vi "Test MQTT-3.1.0-1.vi"(8 "error in (no error)":errorcluster) -> (0 "error out":errorcluster)   [LabVIEW 2013]
uses:
  <vilib>/LabVIEW Open Source Project/MQTT Control Packets/Control Packets/ControlPacket/ControlPacket.lvclass
  <vilib>/addons/_JKI Toolkits/Caraya/classes/Test/Test.lvclass
  <vilib>/addons/_JKI Toolkits/Caraya/classes/Assert/Assert.lvclass
  <vilib>/LabVIEW Open Source Project/MQTT Control Packets/Control Packets/PUBLISH/PUBLISH.lvclass
  <vilib>/LabVIEW Open Source Project/MQTT Connection/MQTT_Connection/Connection/Connection.lvclass
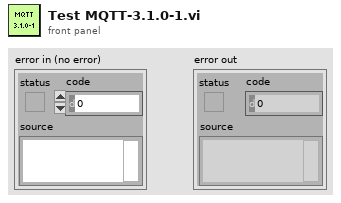
[diagram p1: front panel]
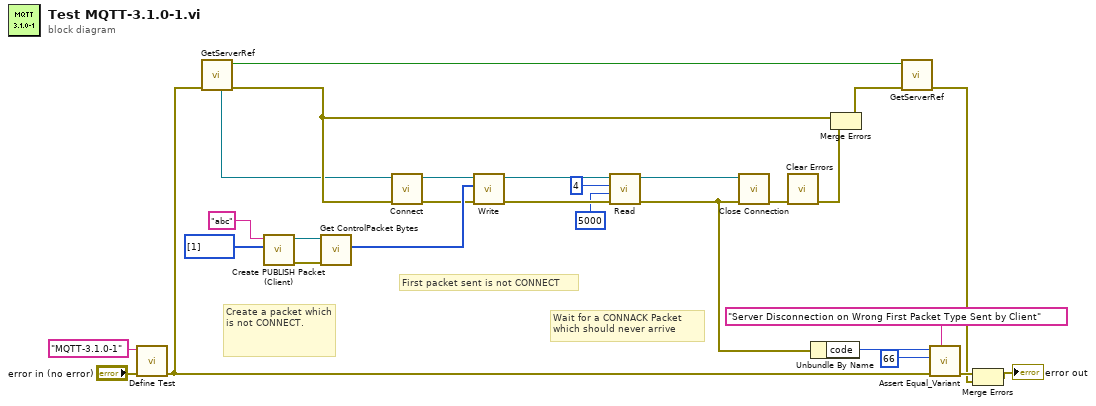
[diagram p0: block diagram]
diagram:
  # "Wait for a CONNACK Packet\nwhich should never arrive"
  # "Create a packet which is not CONNECT."
  # "First packet sent is not CONNECT"
  n1 = call <vilib>:"Define Test.vi"("error in (no error)"="error in (no error)", "Label (VI Title)"="MQTT-3.1.0-1") -> ("error out"=w6:errorcluster)  [unwired: 9 in]
  n2 = call "GetServerRef.vi"("error in"=w6) -> ("error out"=w5:errorcluster, "Created"=w7:bool, "Connection Config"=w2:refnum<class "Connection.lvclass">)  [unwired: 7 in, 1 out]
  n3 = call <vilib>:"Create PUBLISH Packet (Client).vi"("Payload"=u8[] [1], "Topic Name"="abc") -> ("error out"=w12:errorcluster, "PUBLISH"=w13:refnum<class "PUBLISH.lvclass">)  [unwired: 6 in, 2 out]
  n4 = call <vilib>:"Get ControlPacket Bytes.vi"("error in (no error)"=w12, "ControlPacket"=w13) -> ("Bytes Stream"=w14:u8[])  [unwired: 6 in, 3 out]
  n5 = call <vilib>:"Connect.vi"("error in (no error)"=w5, "Connection in"=w2) -> ("error out"=w8:errorcluster, "Connection out"=w9:refnum<class "Connection.lvclass">)  [unwired: 8 in]
  n6 = call <vilib>:"Write.vi"("error in (no error)"=w8, "Bytes"=w14, "Connection in"=w9) -> ("error out"=w27:errorcluster, "Connection"=w28:refnum<class "Connection.lvclass">)  [unwired: 7 in]
  n7 = call <vilib>:"Read.vi"("error in (no error)"=w27, "timeout (2000 ms)"=5000 ("timeout ms (25000)"), "bytes to read (100)"=4 ("bytes to read"), "TCPConnection in"=w28) -> ("error out"=w16:errorcluster, "TCPConnection out"=w26:refnum<class "Connection.lvclass">)  [unwired: 3 in, 3 out]
  n8 = call <vilib>:"Close Connection.vi"("error in (no error)"=w16, "Connection in"=w26) -> ("error out"=w20:errorcluster)  [unwired: 8 in, 1 out]
  n9 = call <vilib>:"Clear Errors.vi"("error in (no error)"=w20) -> ("error out"=w15:errorcluster)  [unwired: 6 in]
  n10 = Unbundle By Name(w16) -> ("code"=w22:i32)
  n11 = Merge Errors(w5, w15) -> (w4:errorcluster)
  n12 = call "GetServerRef.vi"("error in"=w4, "Destroy (F)"=w7) -> ("error out"=w3:errorcluster)  [unwired: 6 in, 3 out]
  n13 = call <vilib>:"Assert Equal_Variant.vi"("Label"="Server Disconnection on Wrong First Packet Type Sent by Client", "error in (no error)"=w6, "Y"=66 ("code"), "X"=w22) -> ("error out"=w25:errorcluster)  [unwired: 7 in]
  n14 = Merge Errors(w25, w3) -> (→"error out":errorcluster)
